vi "Interpret Licor-data.vi"(11 "Licor-data":string[](array[string])) -> (0 "remain":string[](array[string]), 1 "log":string[][](array[string]), 2 "calibration data out":dbl[][](array[numeric]), 3 "source data out":dbl[][](array[numeric]))   [LabVIEW 2010]
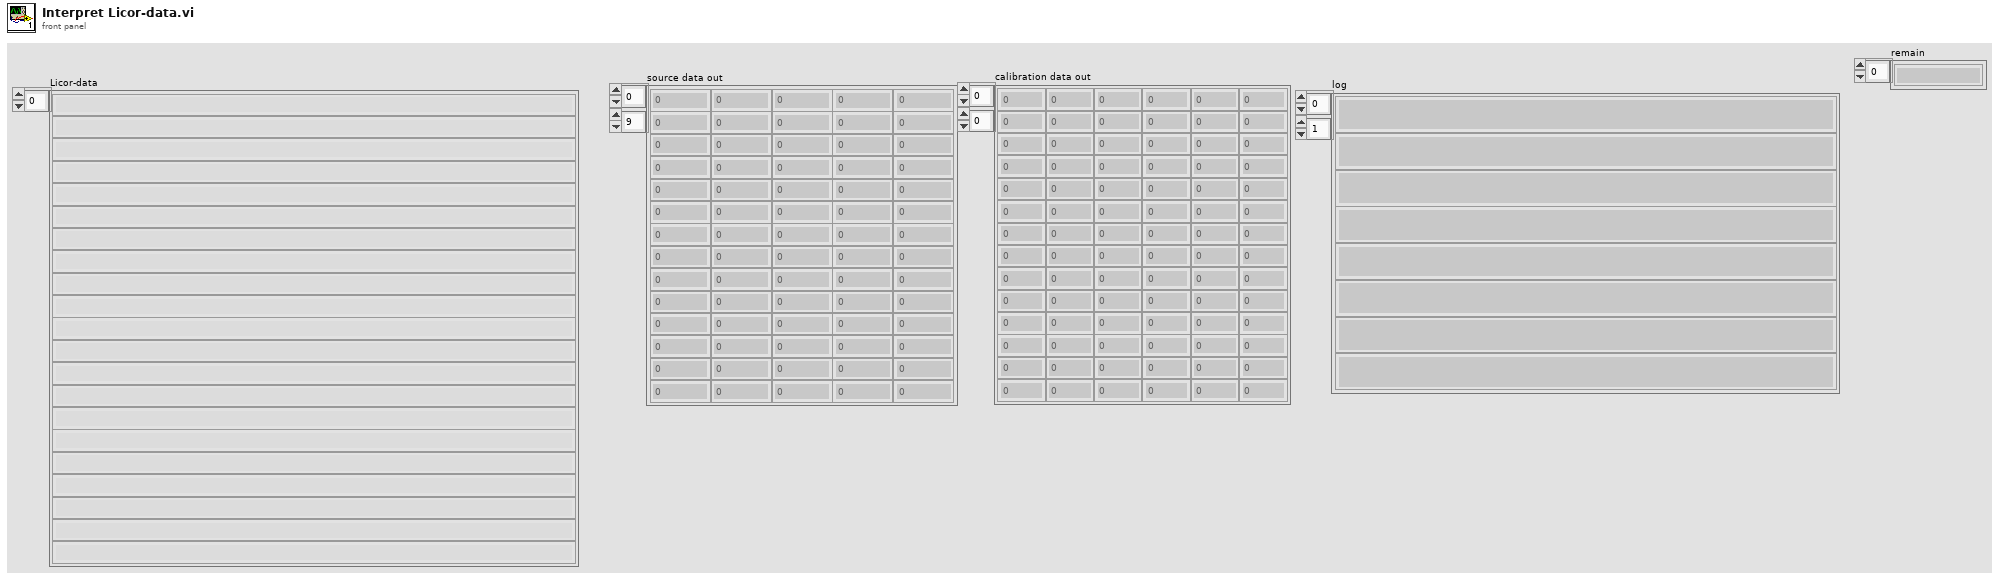
[diagram p1: front panel]
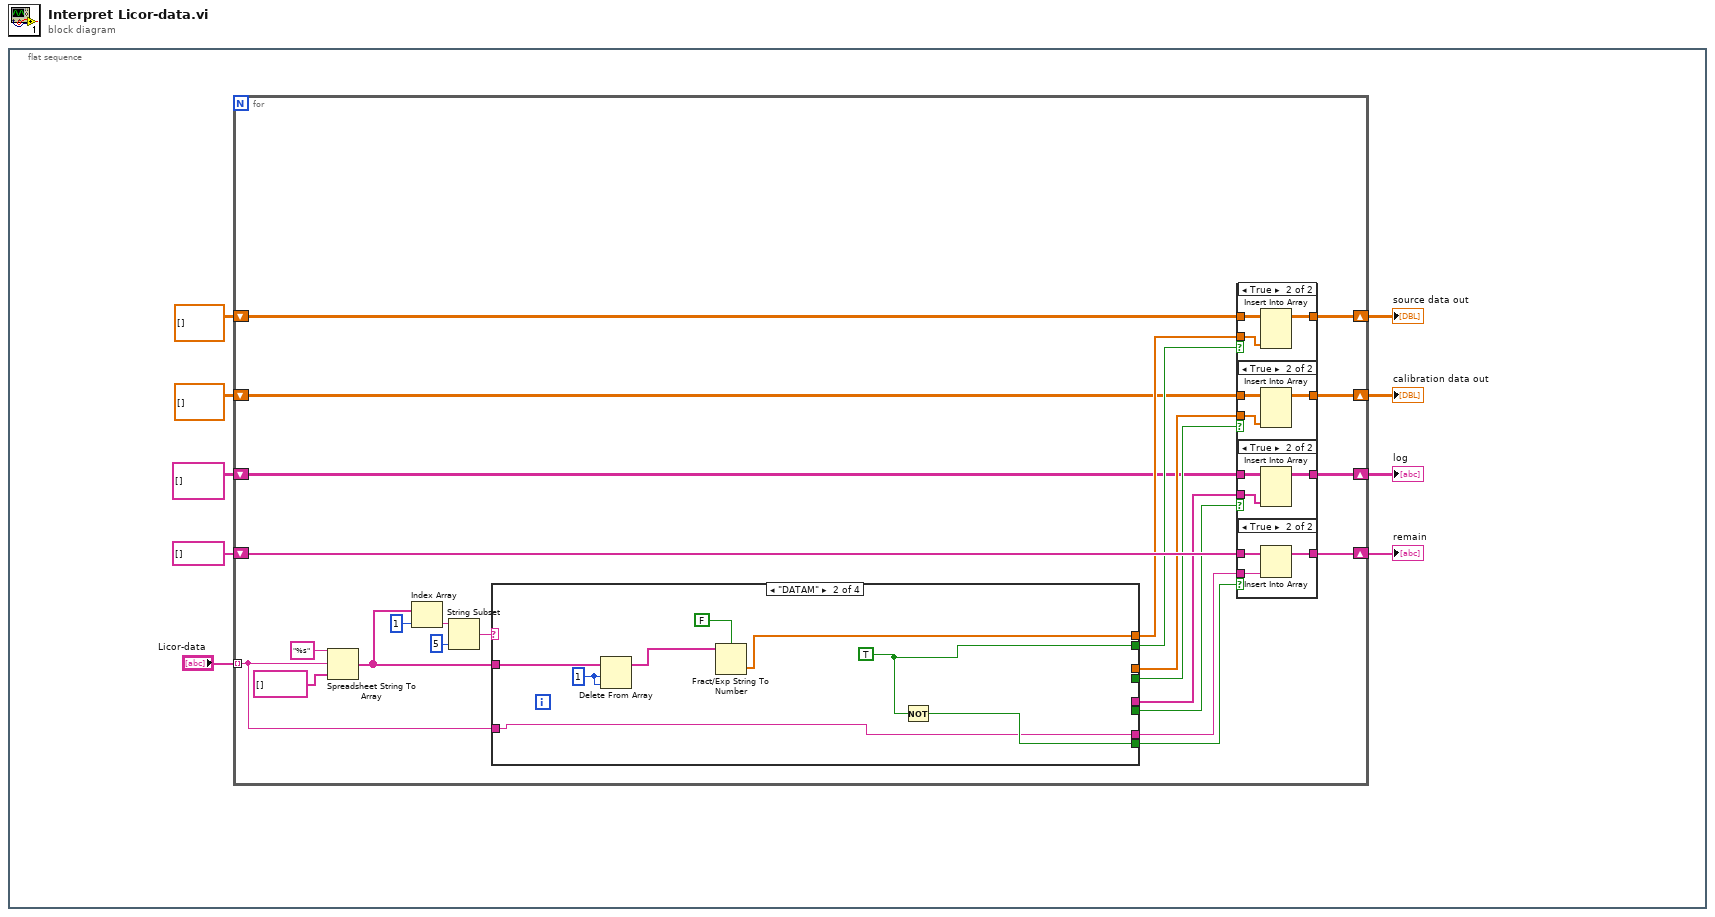
[diagram p0: block diagram]
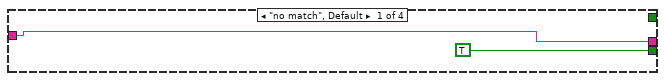
[diagram p6: hidden frame]
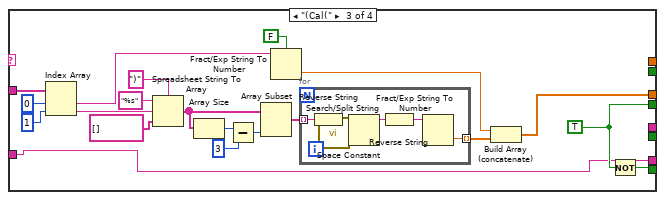
[diagram p7: hidden frame]
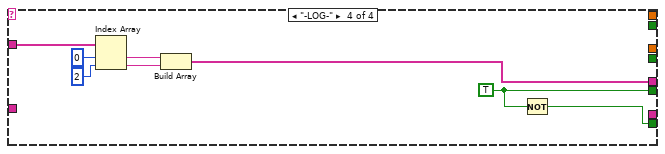
[diagram p8: hidden frame]
diagram:
  n1 = flat-sequence {
    frame #0 {
      n2 = for {
        tunnel: "Licor-data" -> [w26] mode=indexing
        shift-right: [w23] -> w1
        shift-left: string[] [] -> [w22]
        shift-right: [w15] -> w2
        shift-left: string[][] [] -> [w10]
        shift-right: [w14] -> w3
        shift-left: dbl[][] [] -> [w11]
        shift-right: [w13] -> w8
        shift-left: dbl[][] [] -> [w12]
        n3 = Spreadsheet String To Array(format string="%s", spreadsheet string=w26, array type (2D Dbl)=string[] []) -> (array=w27:string[])  [unwired: 1 in]
        n4 = Index Array(array=w27, index=1 ("Index")) -> (element=w30:string)
        n5 = String Subset(string=w30, length (rest)=5 ("Länge (Rest)")) -> (substring=w32:string)  [unwired: 1 in]
        n6 = case shown="\"DATAM\"" w32 {
          tunnel: [_ _ w66 _] -> w18
          tunnel: [_ w52 _ _] -> w16
          tunnel: [_ w56 _ _] -> w17
          tunnel: [_ _ w64 _] -> w19
          tunnel: w27 -> [_ w59 w70 w91]
          tunnel: [_ _ _ w88] -> w20
          tunnel: [w50 w55 w63 _] -> w24
          tunnel: [_ _ _ w87] -> w21
          tunnel: [TRUE w57 w65 w86] -> w25
          tunnel: w26 -> [w50 w55 w63 _]
          frame "no match", Default {
          }
          frame "DATAM" {
            w56 = TRUE
            w58 = 1 ("Länge")
            n7 = Delete From Array(array=w59, length=w58, index=w58) -> (array with subset deleted=w54:string[])  [unwired: 1 out]
            n8 = Fract/Exp String To Number(use system decimal point (T)=FALSE ("Systemdezimalzeichen verwenden (T)"), string=w54) -> (number=w52:dbl[])  [unwired: 2 in, 1 out]
            n9 = Not(x=w56) -> (.not. x?=w57:bool)
          }
          frame "(Cal(" {
            w64 = TRUE
            n10 = Index Array(array=w70, index #1=0 ("Index"), index #2=1 ("Index")) -> (element #1=w62:string, element #2=w67:string)
            n11 = Spreadsheet String To Array(delimiter (Tab)=")" ("Trennzeichen (Tabulator)"), format string="%s" ("Format-String"), spreadsheet string=w67, array type (2D Dbl)=string[] []) -> (array=w75:string[])
            n12 = Array Size(array=w75) -> (size(s)=w76:i32)
            n13 = Subtract(x=w76, y=3) -> (x-y=w78:i32)
            n14 = Array Subset(array=w75, length=w78) -> (w79:string[])  [unwired: 1 in]
            n15 = Fract/Exp String To Number(use system decimal point (T)=FALSE ("Systemdezimalzeichen verwenden (T)"), string=w62) -> (number=w61:dbl)  [unwired: 2 in, 1 out]
            n16 = for {
              tunnel: w79 -> [w83] mode=indexing
              tunnel: [w84] -> w71 mode=indexing
              n17 = Reverse String(1:w83) -> (0:w82:string)
              n18 = call <vilib>:"Space Constant.vi"() -> ("String"=w85:string)
              n19 = Search/Split String(string=w82, search string/char (-)=w85) -> (substring before match=w81:string)  [unwired: 1 in, 2 out]
              n20 = Reverse String(1:w81) -> (0:w80:string)
              n21 = Fract/Exp String To Number(string=w80) -> (number=w84:dbl)  [unwired: 3 in, 1 out]
            }
            n22 = Build Array (concatenate)(w61, w71) -> (w66:dbl[])
            n23 = Not(x=w64) -> (.not. x?=w65:bool)
          }
          frame "-LOG-" {
            w87 = TRUE
            n24 = Index Array(array=w91, index #1=0 ("Index"), index #2=2 ("Index")) -> (element #1=w90:string, element #2=w89:string)
            n25 = Build Array(w90, w89) -> (w88:string[])
            n26 = Not(x=w87) -> (.not. x?=w86:bool)
          }
        }
        n27 = case shown="True" w17 {
          tunnel: w16 -> [_ w49]
          tunnel: [w46 w48] -> w13
          tunnel: w12 -> [w46 w47]
          frame False {
          }
          frame True {
            n28 = Insert Into Array(array=w47, new element=w49) -> (w48:dbl[][])  [unwired: 2 in]
          }
        }
        n29 = case shown="True" w19 {
          tunnel: w18 -> [_ w45]
          tunnel: [w42 w44] -> w14
          tunnel: w11 -> [w42 w43]
          frame False {
          }
          frame True {
            n30 = Insert Into Array(array=w43, new element=w45) -> (w44:dbl[][])  [unwired: 2 in]
          }
        }
        n31 = case shown="True" w21 {
          tunnel: w20 -> [_ w41]
          tunnel: [w38 w40] -> w15
          tunnel: w10 -> [w38 w39]
          frame False {
          }
          frame True {
            n32 = Insert Into Array(array=w39, new element=w41) -> (w40:string[][])  [unwired: 2 in]
          }
        }
        n33 = case shown="True" w25 {
          tunnel: w24 -> [_ w37]
          tunnel: [w34 w36] -> w23
          tunnel: w22 -> [w34 w35]
          frame False {
          }
          frame True {
            n34 = Insert Into Array(array=w35, new element=w37) -> (w36:string[])  [unwired: 1 in]
          }
        }
      }
      "calibration data out" <- w3
      "source data out" <- w8
      "log" <- w2
      "remain" <- w1
    }
  }
